vi "LEBITplc.PubMonServices.vi"(0 "i ref in":refnum<vi>, 2 "i attribute in":T1, 5 "error in":errorcluster) -> (14 "i ref out":refnum<vi>, 16 "i attribute out":T1, 17 "MonValueServiceID":i32[](array[numeric]), 19 "error out":errorcluster)   [LabVIEW 2014, in "LEBITplc.lvlib"]
uses:
  LEBITplc.lvlib
  LEBITplc.i attribute.ctl
  CSlibraries/UtilityLib/UtilityLib.valueStatus.ctl
  CSlibraries/UtilityLib/UtilityLib.lvlib
  CS_Core/CSSystem/CoreLib/CoreLib.lvlib
  CSlibraries-extern/DimLVEvent/LVDimInterface/LVDimInterface.lvlib
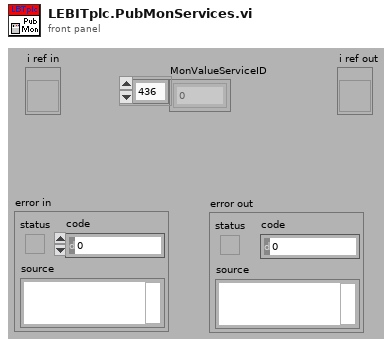
[diagram p1: front panel]
types:
  T1 = typedef "LEBITplc.lvlib/LEBITplc.i attribute.ctl" = cluster{"LLFLocation":string, "SetFileLocation":string, "nickNames":string[], "setValuePLCServiceID":i32[], "GUIServiceID":i32[], "monValuePLC":string[], "SetValueServiceID":i32[], "MonValueServiceID":i32[], "SetValue":dbl[][], "SetValueMin":dbl[], "SetValueMax":dbl[], "SetValueInfoServiceID":i32[], "GUINames":string[], "ListOfBases":string[], "Scale":dbl[], "Offset":dbl[], "setValuePLC":string[], "BaseName":string[], "ScaleServiceID":i32[], "OffsetServiceID":i32[], "AllPLCValues":string[], "CondSpecialArray":string[][], "CondSpecialIndex":i32[], "CondSpecialMonValue":dbl[], "RecentlyChanged":i32[], "SetFileLocationID":i32, "Dependent-Monitors":string[][], "LastLoadedFiles":string[], "IonGuideCalibLocation":string, "Monitor Dependent":string[], "Special":string[], "PLC?":bool[], "Start Date":string, "ListOfBasesServiceID":i32, "SETRA VISA resource":refnum<visa-resource-name>}
  T2 = typedef "UtilityLib.lvlib/UtilityLib.valueStatus.ctl" = enum16{"no info available", "stand by/off", "on", "warning", "alarm/malfunction", "not implemented", "user action required", "important information", "system default", "control default", "indicator default", "button default"}
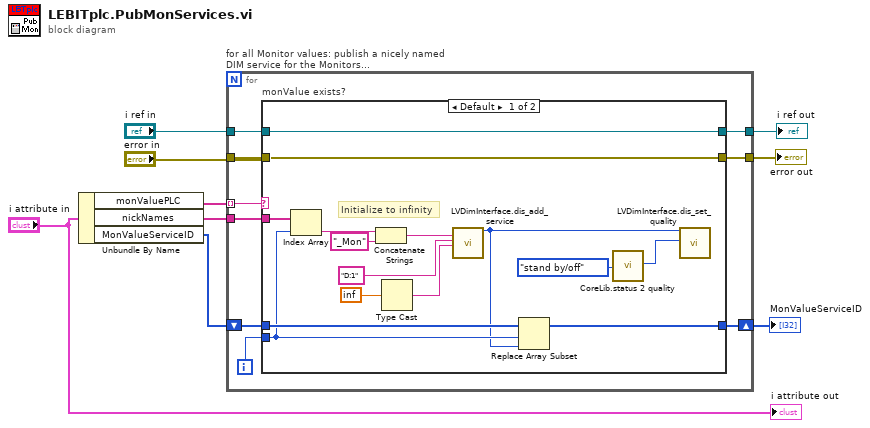
[diagram p0: block diagram]
diagram:
  n1 = Unbundle By Name("i attribute in") -> ("monValuePLC"=w1:string[], "nickNames"=w4:string[], "MonValueServiceID"=w5:i32[])
  n2 = for "for all Monitor values: publish a nicely named DIM service for the Monitors..." {
    tunnel: w1 -> [w18] mode=indexing
    tunnel: w4 -> [w17]
    shift-right: [w14] -> w8
    shift-left: w5 -> [w15]
    tunnel: "i ref in" -> [w13]
    tunnel: "error in" -> [w12]
    tunnel: [w11] -> w7
    tunnel: [w10] -> w6
    i -> [w16]
    n3 = case "monValue exists?" shown="Default" w18 {
      tunnel: w17 -> [w31 _]
      tunnel: w16 -> [w28 _]
      tunnel: w15 -> [w29 w36]
      tunnel: [w27 w36] -> w14
      tunnel: w13 -> [w20 w35]
      tunnel: w12 -> [w19 w34]
      tunnel: [w19 w34] -> w11
      tunnel: [w20 w35] -> w10
      frame Default {
        # "Initialize to infinity"
        n4 = Index Array(array=w31, index=w28) -> (element=w26:string)
        n5 = Concatenate Strings(w26, "_Mon" ("string")) -> (w32:string)
        n6 = Type Cast(x=inf) -> (*(type *) &x=w30:string)  [unwired: 1 in]
        n7 = call "LVDimInterface.dis_add_service.vi"("serviceName"=w32, "typeDescriptor"="D:1", "data"=w30) -> ("my_serviceID"=w22:i32)  [unwired: 15 in, 1 out]
        n8 = Replace Array Subset(array=w29, new element=w22, index=w28) -> (w27:i32[])
        n9 = call "CoreLib.status 2 quality.vi"("valueStatus"=UtilityLib.valueStatus."stand by/off") -> ("quality"=w24:i32)  [unwired: 18 in]
        n10 = call "LVDimInterface.dis_set_quality.vi"("my_serviceID"=w22, "quality"=w24) -> ()  [unwired: 16 in, 2 out]
      }
      frame "" {
      }
    }
  }
  "MonValueServiceID" <- w8
  "error out" <- w7
  "i ref out" <- w6
  "i attribute out" <- "i attribute in"
